vi "Write_conversion-formula.vi"(8 "error in (no error)":errorcluster, 10 "conversion formula":string, 11 "PrepLineObject in":refnum<class "PrepLineObject.lvclass">) -> (0 "error out":errorcluster, 3 "PrepLineObject out":refnum<class "PrepLineObject.lvclass">)   [LabVIEW 2018, in "PrepLineObject.lvclass"]
uses:
  PrepLineObject.lvclass
  PrepLineObject.lvclass/PrepLineObject.ctl
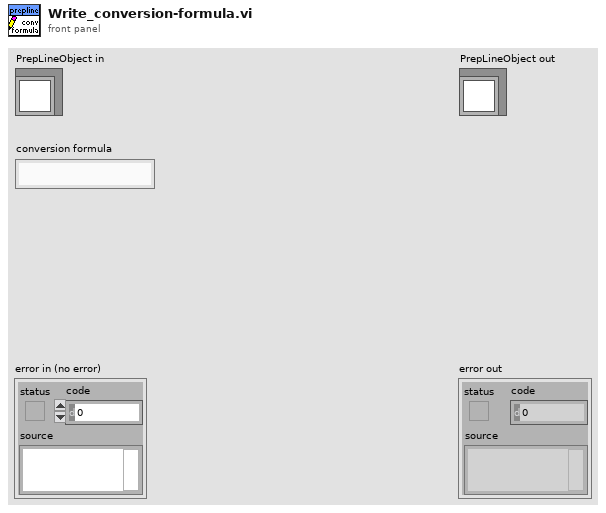
[diagram p1: front panel]
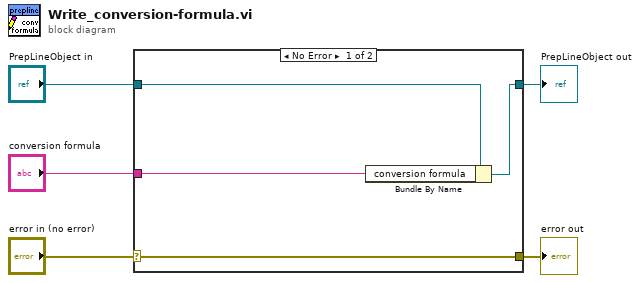
[diagram p0: block diagram]
diagram:
  n1 = case shown="No Error" "error in (no error)" {
    selector: "error in (no error)" -> [w9 w10]
    tunnel: [w9 w10] -> w4
    tunnel: [w7 w11] -> w2
    tunnel: "PrepLineObject in" -> [w8 w11]
    tunnel: "conversion formula" -> [w6 _]
    frame No Error {
      n2 = Bundle By Name(cluster=w8, "conversion formula"=w6) -> (w7:refnum<class "PrepLineObject.lvclass">)
    }
    frame Error {
    }
  }
  "error out" <- w4
  "PrepLineObject out" <- w2
